vi "set_points.vi"(7 "mode":T1, 8 "error in (no error)":errorcluster, 10 "points (dimensions/points)":dbl[][](array[numeric]), 11 "PointCollection in":refnum<class "PointCollection.lvclass">) -> (0 "error out":errorcluster, 3 "PointCollection out":refnum<class "PointCollection.lvclass">)   [LabVIEW 2010, in "PointCollection.lvclass"]
uses:
  PointCollection.lvclass
  mode_enum.ctl
  PointCollection.lvclass/PointCollection.ctl
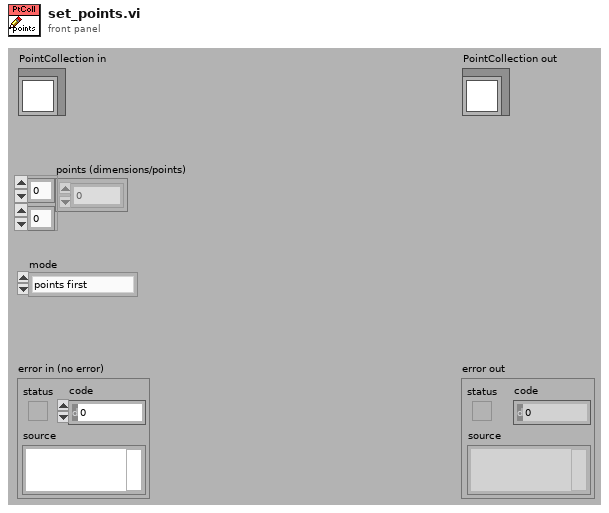
[diagram p1: front panel]
types:
  T1 = typedef "PointCollection.lvclass/mode_enum.ctl" = enum16{"points first", "dimensions first"}
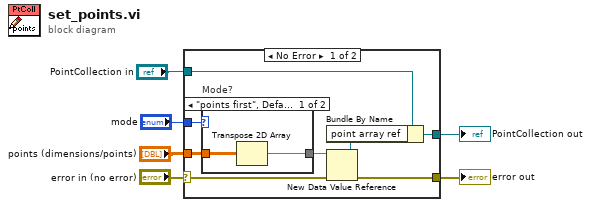
[diagram p0: block diagram]
diagram:
  n1 = case shown="No Error" "error in (no error)" {
    selector: "error in (no error)" -> [w14 w19]
    tunnel: [w7 w19] -> w5
    tunnel: [w11 w18] -> w3
    tunnel: "PointCollection in" -> [w12 w18]
    tunnel: "points (dimensions/points)" -> [w10 _]
    tunnel: "mode" -> [w8 _]
    frame No Error {
      n2 = case "Mode?" shown="\"points first\", Default" w8 {
        tunnel: w10 -> [w16 w17]
        tunnel: [w15 w17] -> w9
        frame "points first", Default {
          n3 = Transpose 2D Array(2D array=w16) -> (transposed array=w15:dbl[][])
        }
        frame "dimensions first" {
        }
      }
      n4 = New Data Value Reference(data value=w9, error in=w14) -> (data value reference=w13:refnum<data-value>, error out=w7:errorcluster)
      n5 = Bundle By Name(cluster=w12, "point array ref"=w13) -> (w11:refnum<class "PointCollection.lvclass">)
    }
    frame Error {
    }
  }
  "error out" <- w5
  "PointCollection out" <- w3
